vi "MatchCarexToEMG.vi"(8 "EMGFileList":string[](array[string]), 11 "CarexFileName":string) -> (0 "FileNameIndex":i32, 3 "MatchedFileName":string)   [LabVIEW 2016]
panel:
  out "spreadsheet string":string
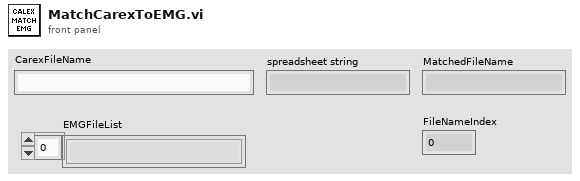
[diagram p1: front panel]
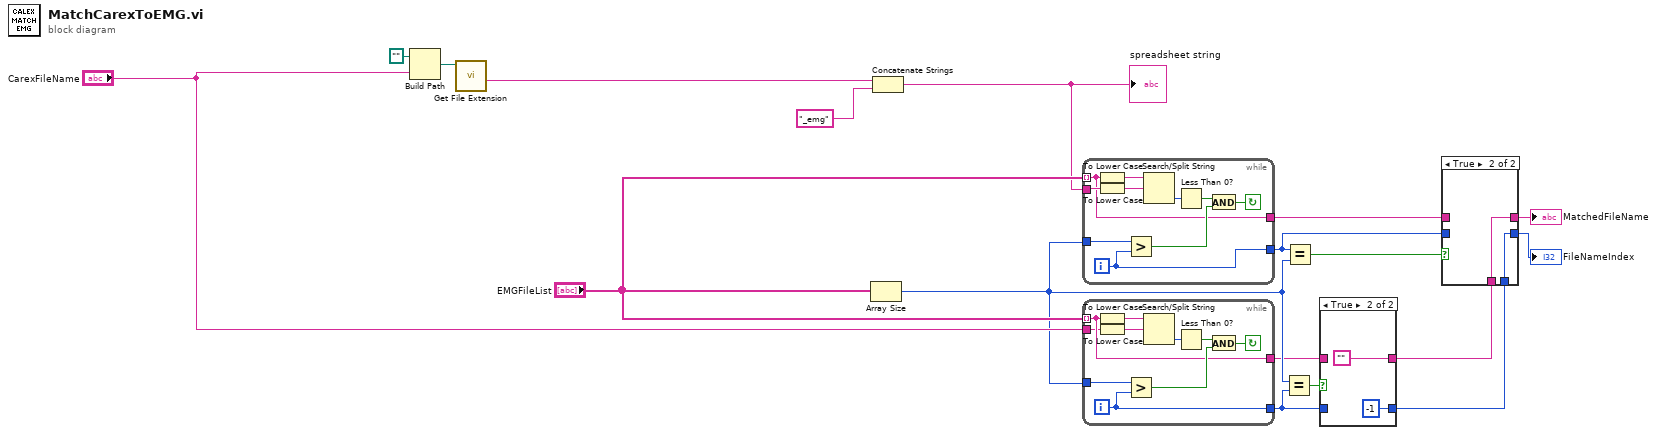
[diagram p0: block diagram]
diagram:
  n1 = Build Path(base path=path "", name or relative path="CarexFileName") -> (appended path=w12:path)
  n2 = call <vilib>:"Get File Extension.vi"("file"=w12) -> ("filename without extension"=w3:string)  [unwired: 6 in, 4 out]
  n3 = Array Size(array="EMGFileList") -> (size(s)=w8:i32)
  n4 = Concatenate Strings(w3, "_emg" ("string")) -> (w2:string)
  "spreadsheet string" <- w2
  n5 = while {
    tunnel: "EMGFileList" -> [w19] mode=indexing
    tunnel: w2 -> [w25]
    tunnel: [w19] -> w17
    tunnel: [w24] -> w16
    tunnel: w8 -> [w23]
    i -> [w24]
    stop <- w20 continue-if-true
    n6 = To Lower Case(string=w19) -> (all lower case string=w28:string)
    n7 = To Lower Case(string=w25) -> (all lower case string=w26:string)
    n8 = Greater?(x=w23, y=w24) -> (0:w21:bool)
    n9 = Search/Split String(string=w28, search string/char (-)=w26) -> (offset of match=w27:i32)  [unwired: 1 in, 2 out]
    n10 = Less Than 0?(x=w27) -> (x < 0?=w22:bool)
    n11 = And(x=w22, y=w21) -> (x .and. y?=w20:bool)
  }
  n12 = while {
    tunnel: "EMGFileList" -> [w30] mode=indexing
    tunnel: [w30] -> w7
    tunnel: [w35] -> w4
    tunnel: w8 -> [w34]
    tunnel: "CarexFileName" -> [w29]
    i -> [w35]
    stop <- w31 continue-if-true
    n13 = To Lower Case(string=w30) -> (all lower case string=w38:string)
    n14 = To Lower Case(string=w29) -> (all lower case string=w36:string)
    n15 = Greater?(x=w34, y=w35) -> (0:w32:bool)
    n16 = Search/Split String(string=w38, search string/char (-)=w36) -> (offset of match=w37:i32)  [unwired: 1 in, 2 out]
    n17 = Less Than 0?(x=w37) -> (x < 0?=w33:bool)
    n18 = And(x=w33, y=w32) -> (x .and. y?=w31:bool)
  }
  n19 = Equal?(x=w8, y=w4) -> (x = y?=w9:bool)
  n20 = Equal?(x=w16, y=w8) -> (x = y?=w18:bool)
  n21 = case shown="True" w9 {
    tunnel: w7 -> [w40 _]
    tunnel: [w40 ""] -> w6
    tunnel: [w39 -1] -> w5
    tunnel: w4 -> [w39 _]
    frame False {
    }
    frame True {
    }
  }
  n22 = case shown="True" w18 {
    tunnel: w17 -> [w44 _]
    tunnel: w16 -> [w43 _]
    tunnel: [w44 w46] -> w15
    tunnel: [w43 w45] -> w14
    tunnel: w6 -> [_ w46]
    tunnel: w5 -> [_ w45]
    frame False {
    }
    frame True {
    }
  }
  "MatchedFileName" <- w15
  "FileNameIndex" <- w14
